vi "fronts64_ext.vi"(5 "NOT IN OLD":u64 format="%x", 7 "IN":u64 format="%x") -> (1 "NOT IN":u64 format="%x", 2 "FALL":u64 format="%x", 3 "RAISE":u64 format="%x")   [LabVIEW 2019, in "Logik.lvlib"]
uses:
  Logik.lvlib
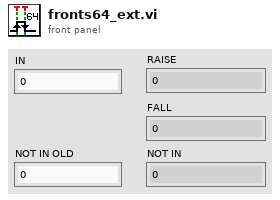
[diagram p1: front panel]
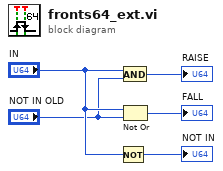
[diagram p0: block diagram]
diagram:
  n1 = Not(x="IN") -> (.not. x?=→"NOT IN":u64)
  n2 = And(x="IN", y="NOT IN OLD") -> (x .and. y?=→"RAISE":u64)
  n3 = Not Or(1:"NOT IN OLD", 2:"IN") -> (0:→"FALL":u64)
